vi "Stage 3.5 Placing GUI into subVIs.vi"() -> ()   [LabVIEW 2020]
uses:
  HRM-Stage3-User_events.ctl
  HRM-Stage3-init_cluster.ctl
panel:
  out "Process Error":errorcluster
  out "error out":errorcluster
  out "error out Hardware":errorcluster
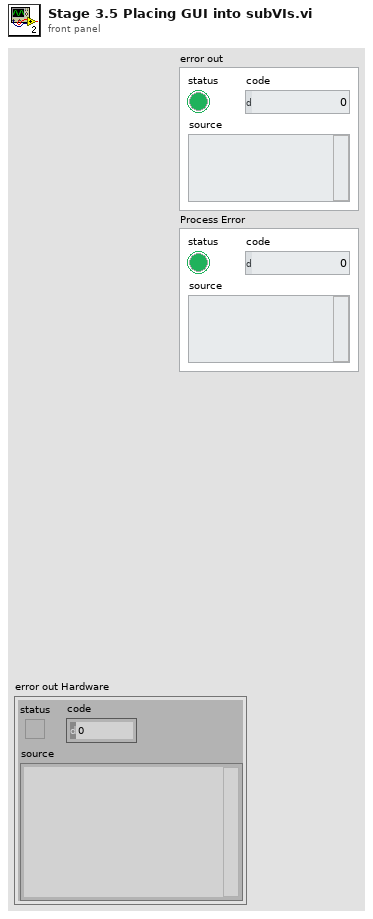
[diagram p1: front panel]
types:
  T1 = typedef "HRM-Stage3-init_cluster.ctl" = cluster{"User events":T2}
  T2 = typedef "HRM-Stage3-User_events.ctl" = cluster{"Signal to remove":refnum<user-event>, "Sample size":refnum<user-event>, "Filtered wf":refnum<user-event>, "Unfiltered wf":refnum<user-event>, "Raw wf":refnum<user-event>, "Pulse":refnum<user-event>, "Stop":refnum<user-event>}
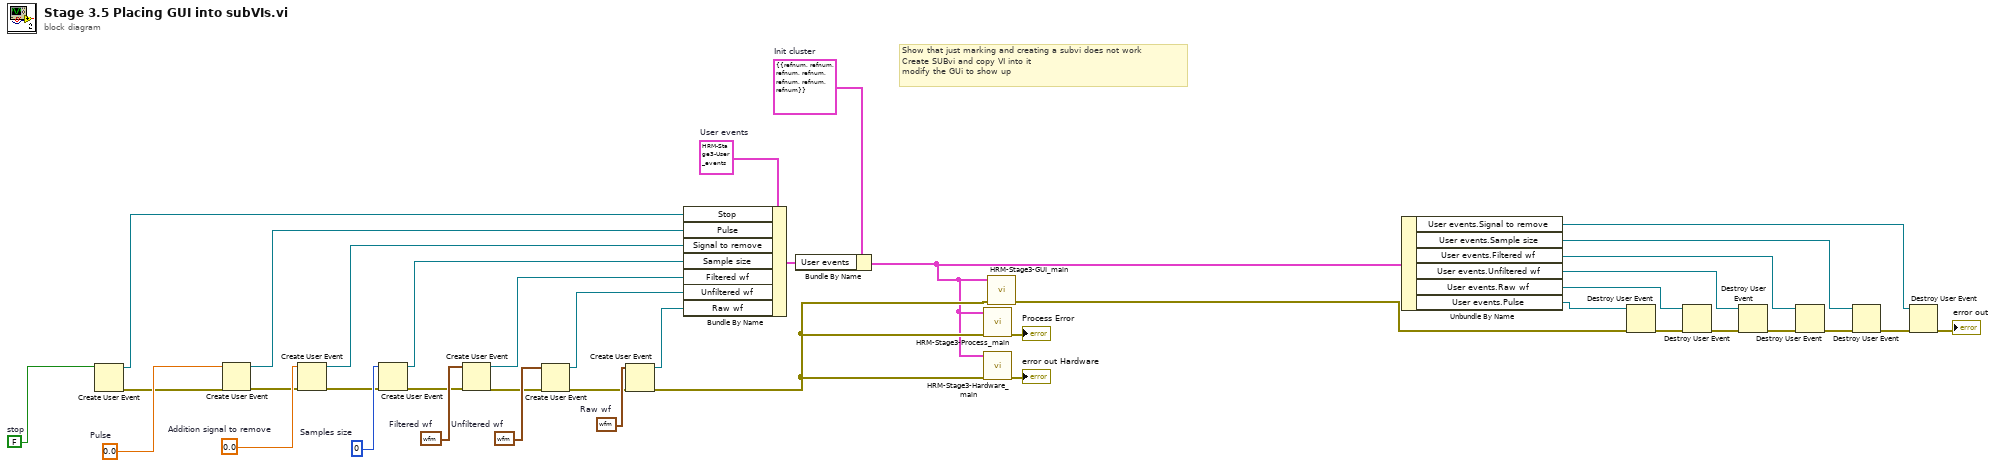
[diagram p0: block diagram]
diagram:
  w18 = FALSE  # stop
  w20 = T1 {"User events"={"Signal to remove"=refnum, "Sample size"=refnum, "Filtered wf"=refnum, "Unfiltered wf"=refnum, "Raw wf"=refnum, "Pulse"=refnum, "Stop"=refnum}}  # Init cluster
  w23 = 0.0  # Pulse
  w29 = T2 {"Signal to remove"=refnum, "Sample size"=refnum, "Filtered wf"=refnum, "Unfiltered wf"=refnum, "Raw wf"=refnum, "Pulse"=refnum, "Stop"=refnum}  # User events
  w34 = 0  # Samples size
  w35 = 0.0  # Addition signal to remove
  w36 = waveform(dbl) {"t0"=timestamp(0 s since 1904-01-01), "dt"=1.0, "Y"=[]}  # Filtered wf
  w37 = waveform(dbl) {"t0"=timestamp(0 s since 1904-01-01), "dt"=1.0, "Y"=[]}  # Unfiltered wf
  w38 = waveform(dbl) {"t0"=timestamp(0 s since 1904-01-01), "dt"=1.0, "Y"=[]}  # Raw wf
  # "Show that just marking and creating a subvi does not work\nCreate SUBvi and copy VI into it\nmodify the GUi to show up"
  n1 = Create User Event(user event datatype=w18) -> (user event=w16:refnum<user-event>, error out=w17:errorcluster)  [unwired: 1 in]
  n2 = Create User Event(user event datatype=w23, error in=w17) -> (user event=w22:refnum<user-event>, error out=w21:errorcluster)
  n3 = Create User Event(user event datatype=w35, error in=w21) -> (user event=w28:refnum<user-event>, error out=w30:errorcluster)
  n4 = Create User Event(user event datatype=w34, error in=w30) -> (user event=w27:refnum<user-event>, error out=w31:errorcluster)
  n5 = Create User Event(user event datatype=w36, error in=w31) -> (user event=w26:refnum<user-event>, error out=w32:errorcluster)
  n6 = Create User Event(user event datatype=w37, error in=w32) -> (user event=w25:refnum<user-event>, error out=w33:errorcluster)
  n7 = Create User Event(user event datatype=w38, error in=w33) -> (user event=w24:refnum<user-event>, error out=w15:errorcluster)
  n8 = Bundle By Name(cluster=w29, "Stop"=w16, "Pulse"=w22, "Signal to remove"=w28, "Sample size"=w27, "Filtered wf"=w26, "Unfiltered wf"=w25, "Raw wf"=w24) -> (w19:T2)
  n9 = Bundle By Name(cluster=w20, "User events"=w19) -> (w2:T1)
  n10 = call "HRM-Stage3-Process_main.vi"("error in (no error)"=w15, "Init cluster"=w2) -> ("error out"=→"Process Error":errorcluster)  [unwired: 9 in]
  n11 = call "HRM-Stage3-Hardware_main.vi"("error in (no error)"=w15, "Init cluster"=w2) -> ("error out"=→"error out Hardware":errorcluster)  [unwired: 9 in]
  n12 = call "HRM-Stage3-GUI_main.vi"("error in (no error)"=w15, "Init cluster"=w2) -> ("error out"=w3:errorcluster)  [unwired: 9 in]
  n13 = Unbundle By Name(w2) -> ("User events.Signal to remove"=w4:refnum<user-event>, "User events.Sample size"=w5:refnum<user-event>, "User events.Filtered wf"=w6:refnum<user-event>, "User events.Unfiltered wf"=w7:refnum<user-event>, "User events.Raw wf"=w8:refnum<user-event>, "User events.Pulse"=w9:refnum<user-event>)
  n14 = Destroy User Event(user event=w9, error in=w3) -> (error out=w10:errorcluster)
  n15 = Destroy User Event(user event=w8, error in=w10) -> (error out=w14:errorcluster)
  n16 = Destroy User Event(user event=w7, error in=w14) -> (error out=w13:errorcluster)
  n17 = Destroy User Event(user event=w6, error in=w13) -> (error out=w12:errorcluster)
  n18 = Destroy User Event(user event=w5, error in=w12) -> (error out=w11:errorcluster)
  n19 = Destroy User Event(user event=w4, error in=w11) -> (error out=→"error out":errorcluster)
